vi "DriveJoystickAcquire.vi"(6 "Precision Scaler":dbl=2.0 format="%#_13g", 8 "Rotation Joystick Deadband %":dbl, 11 "XY Joystick Deadband %":dbl) -> (0 "Drive Joystick Buttons":bool[](array[boolean]), 3 "Drive Joystick Values":dbl[](array[numeric]))   [LabVIEW 2018]
uses:
  <vilib>/Rock Robotics/WPI/Utilities/WPI_GetSetVariantRefNum.vi
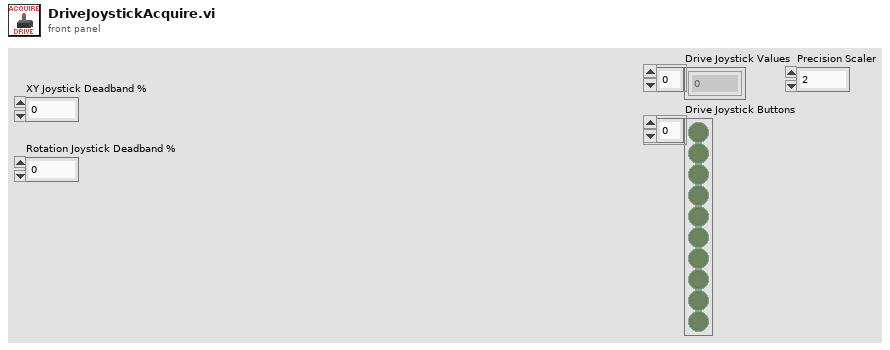
[diagram p1: front panel]
types:
  T1 = typedef "WPI_JoystickDevRef.ctl" = cluster{"Device":T2}
  T2 = typedef "WPI_JoystickDeviceEnum.ctl" = enum16{"USB 0", "USB 1", "USB 2", "USB 3", "USB 4", "USB 5"}
  T3 = typedef "DriveJoystickButtonMapping.ctl" = cluster{"relative encoders?":bool, "zero relative encoder":bool, "reset field orientation":bool, "use field orientation":bool, "braking":bool, "lock rotation":bool, "precision moves":bool}
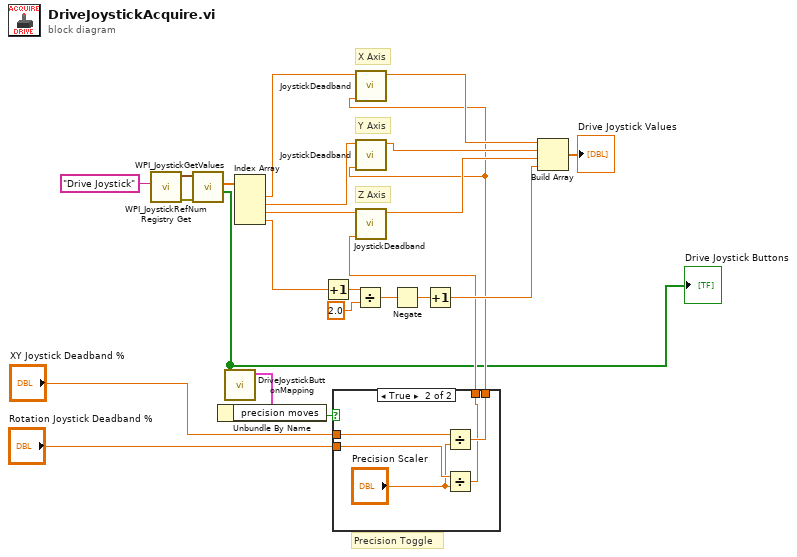
[diagram p0: block diagram]
diagram:
  # "Precision Toggle"
  # "Z Axis"
  # "Y Axis"
  # "X Axis"
  n1 = call <vilib>:"WPI_JoystickRefNum Registry Get.vi"("refnum name"="Drive Joystick") -> ("error out"=w24:errorcluster, "JoystickDevRef"=w23:T1)  [unwired: 9 in]
  n2 = call <vilib>:"WPI_JoystickGetValues.vi"("error in (no error)"=w24, "JoystickDevRef"=w23) -> ("Buttons"=w3:bool[], "Axes"=w21:dbl[])  [unwired: 5 in, 3 out]
  "Drive Joystick Buttons" <- w3
  n3 = call "DriveJoystickButtonMapping.vi"("drive joystick buttons"=w3) -> ("output cluster"=w2:T3)  [unwired: 9 in, 1 out]
  n4 = Unbundle By Name(w2) -> ("precision moves"=w1:bool)
  n5 = Index Array(array=w21) -> (element #1=w20:dbl, element #2=w19:dbl, element #3=w18:dbl, element #4=w15:dbl)  [unwired: 4 in]
  n6 = Increment(x=w15) -> (x+1=w16:dbl)
  n7 = case shown="True" w1 {
    tunnel: "XY Joystick Deadband %" -> [w25 w31]
    tunnel: "Rotation Joystick Deadband %" -> [w26 w30]
    tunnel: [w26 w28] -> w4
    tunnel: [w25 w29] -> w5
    frame False {
    }
    frame True {
      n8 = Divide(x=w31, y="Precision Scaler") -> (x/y=w29:dbl)
      n9 = Divide(x=w30, y="Precision Scaler") -> (x/y=w28:dbl)
    }
  }
  n10 = Divide(x=w16, y=2.0) -> (x/y=w14:dbl)
  n11 = call "JoystickDeadband.vi"("Deadband %"=w5, "Joystick Value"=w20) -> ("Joystick Value"=w9:dbl)  [unwired: 9 in]
  n12 = call "JoystickDeadband.vi"("Deadband %"=w5, "Joystick Value"=w19) -> ("Joystick Value"=w10:dbl)  [unwired: 9 in]
  n13 = call "JoystickDeadband.vi"("Deadband %"=w4, "Joystick Value"=w18) -> ("Joystick Value"=w11:dbl)  [unwired: 9 in]
  n14 = Negate(x=w14) -> (-x=w13:dbl)
  n15 = Increment(x=w13) -> (x+1=w12:dbl)
  n16 = Build Array(w9, w10, w11, w12) -> (→"Drive Joystick Values":dbl[])
